vi "Pointer.Read (1D U8).vi"(8 "error in (no error)":errorcluster, 10 "count":i32, 11 "pointer in":u64) -> (0 "error out":errorcluster, 2 "values":u8[](array[numeric]), 3 "pointer out":u64)   [LabVIEW 2016, in "VeriStand Data.lvlib"]
doc: "Reads a number of values, specified by <B>count</B>, from the provided <B>pointer</B>."
uses:
  VeriStand Data.lvlib
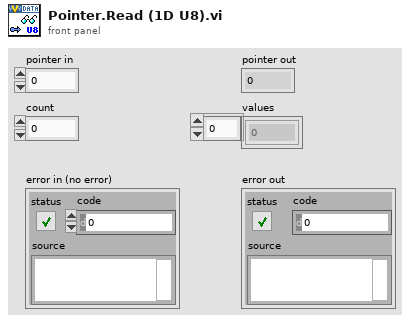
[diagram p1: front panel]
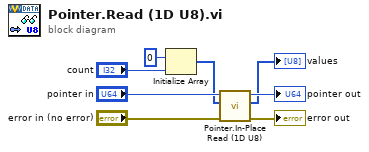
[diagram p0: block diagram]
diagram:
  n1 = Initialize Array(u8 0 ("element"), "count") -> (w1:u8[])
  n2 = call "Pointer.In-Place Read (1D U8).vi"("error in (no error)"="error in (no error)", "allocated array in"=w1, "pointer in"="pointer in") -> ("error out"=→"error out":errorcluster, "array out"=→"values":u8[], "pointer out"=→"pointer out":u64)  [unwired: 6 in]
